vi "motor_contoll.vi"(1 "On/Off":bool, 2 "Enable/Disable":bool, 3 "Forward/Backward":bool) -> (0 "State":bool[](array[boolean]))   [LabVIEW 2017]
uses:
  <vilib>/myRIO/Instrument Drivers/Onboard IO/DIO/typedefs/DIO Reference.ctl
  <vilib>/myRIO/Common/Instrument Driver Framework/Utilities/typedefs/myRIO Generic Hardware Reference.ctl
  <vilib>/myRIO/Common/Instrument Driver Framework/Utilities/typedefs/Hardware Version Enum.ctl
  <vilib>/myRIO/Common/Instrument Driver Framework/Utilities/typedefs/myRIO v1.0 Reference.ctl
  <vilib>/myRIO/Common/Instrument Driver Framework/Utilities/typedefs/Generic FPGA Reference.ctl
  <vilib>/myRIO/Common/Instrument Driver Framework/myRIO v1.0/DIO/typedefs/DIO Channels List.ctl
  <vilib>/myRIO/Common/Instrument Driver Framework/myRIO v1.0/DIO/typedefs/DIO Channels Enum.ctl
  <vilib>/userdefined/High Color/nirio_resource_hc.ctl
  <vilib>/myRIO/Common/Instrument Driver Framework/Utilities/vis/Is FPGA Ref Available.vi
  <vilib>/myRIO/Common/Instrument Driver Framework/myRIO v1.0/DIO/vis/myRIO v1.1 Open DIO.vi
  <vilib>/myRIO/Instrument Drivers/Onboard IO/DIO/vis/Write.vi
  <vilib>/myRIO/Common/Instrument Driver Framework/Utilities/vis/Validate Channels.vi
  <vilib>/myRIO/Common/Instrument Driver Framework/myRIO v1.0/DIO/vis/myRIO v1.0 Reserve DIO.vi
  <vilib>/myRIO/Common/Instrument Driver Framework/myRIO v1.0/Resource Manager/vis/myRIO v1.0 Reserve Channel List.vi
  <vilib>/myRIO/Common/Instrument Driver Framework/myRIO v1.0/DIO/vis/myRIO v1.0 Build MUX Configuration DIO.vi
  <vilib>/myRIO/Common/Instrument Driver Framework/myRIO v1.0/Resource Manager/vis/myRIO v1.0 Reserve Channel.vi
  <vilib>/myRIO/Common/Instrument Driver Framework/myRIO v1.0/Resource Manager/vis/myRIO v1.0 Unreserve Channel.vi
  <vilib>/myRIO/Common/Instrument Driver Framework/myRIO v1.0/Resource Manager/vis/myRIO v1.0 Create Configuration List.vi
  <vilib>/myRIO/Common/Instrument Driver Framework/myRIO v1.0/Resource Manager/vis/myRIO v1.0 Build Mutex Name.vi
  <vilib>/Utility/VariantDataType/GetNumericInfo.vi
  <vilib>/Utility/error.llb/Error Cluster From Error Code.vi
  <vilib>/myRIO/Common/Instrument Driver Framework/myRIO v1.0/myRIO v1.1 Open.vi
  <vilib>/myRIO/Common/Instrument Driver Framework/Utilities/vis/IO Manager.vi
  <vilib>/myRIO/Common/Instrument Driver Framework/Utilities/vis/Configuration Manager.vi
  <vilib>/myRIO/Common/Instrument Driver Framework/myRIO v1.0/Resource Manager/vis/myRIO v1.0 Configure IO.vi
  <vilib>/myRIO/Common/Instrument Driver Framework/myRIO v1.0/myRIO v1.0 Close.vi
  <vilib>/myRIO/Common/Instrument Driver Framework/myRIO v1.0/DIO/vis/myRIO v1.0 Write DIO.vi
  <vilib>/myRIO/Express VI/Onboard Devices/LED/LED Express VI.xnode
  <vilib>/myRIO/Instrument Drivers/Onboard IO/DIO/vis/myRIO DIO Open.xnode
  <vilib>/myRIO/Express VI/Onboard IO/DO/DO Express VI.xnode
  <vilib>/myRIO/Instrument Drivers/Onboard IO/DIO/DIO.lvlib
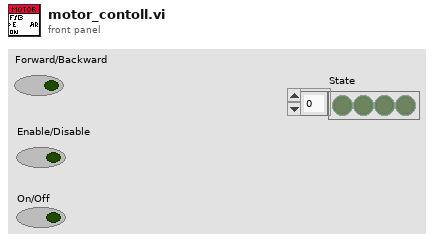
[diagram p1: front panel]
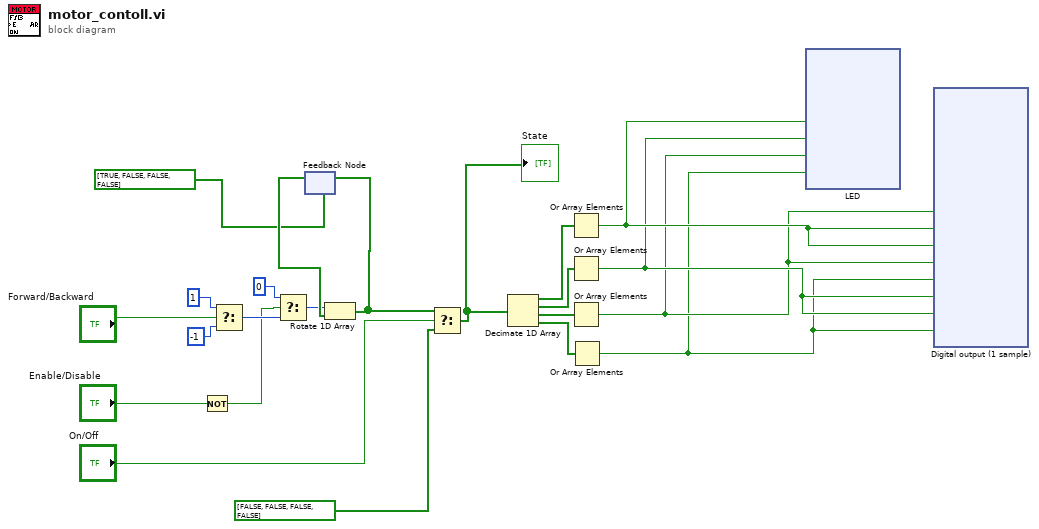
[diagram p0: block diagram]
diagram:
  n1 = Not(x="Enable/Disable") -> (.not. x?=w1:bool)
  n2 = Select(t=1, s="Forward/Backward", f=-1) -> (s? t:f=w19:i32)
  n3 = Select(t=0, s=w1, f=w19) -> (s? t:f=w17:i32)
  n4 = feedback #1(bool[] [TRUE, FALSE, FALSE, FALSE]) -> (w22:bool[])
  n5 = Rotate 1D Array(1:w22, 2:w17) -> (0:w8:bool[])
  n6 = feedback-in #1(w8) -> ()
  n7 = Select(t=w8, s="On/Off", f=bool[] [FALSE, FALSE, FALSE, FALSE]) -> (s? t:f=w4:bool[])
  "State" <- w4
  n8 = Decimate 1D Array(w4) -> (w16:bool[], w15:bool[], w14:bool[], w13:bool[])
  n9 = Or Array Elements(Boolean array=w16) -> (logical OR=w12:bool)
  n10 = Or Array Elements(Boolean array=w15) -> (logical OR=w11:bool)
  n11 = Or Array Elements(Boolean array=w14) -> (logical OR=w10:bool)
  n12 = Or Array Elements(Boolean array=w13) -> (logical OR=w9:bool)
  n13 = xnode "LED"("LED0"=w12, "LED1"=w11, "LED2"=w10, "LED3"=w9) -> ()  [unwired: 1 in, 1 out]
  n14 = xnode "Digital output (1 sample)"("C/DIO0 (DIO0)"=w10, "C/DIO1 (DIO1)"=w12, "C/DIO2 (DIO2)"=w12, "C/DIO3 (DIO3)"=w10, "C/DIO4 (DIO4)"=w9, "C/DIO5 (DIO5)"=w11, "C/DIO6 (DIO6)"=w11, "C/DIO7 (DIO7)"=w9) -> ()  [unwired: 1 in, 1 out]
